vi "String - Format to (HH_colon_MM).vi"(10 "upper limit (Default 23 Hours)":i32=23, 11 "xx:xx":string) -> (2 "seconds":dbl format="%<%H:%M>t", 3 "(HH:mm)":string)   [LabVIEW 2013]
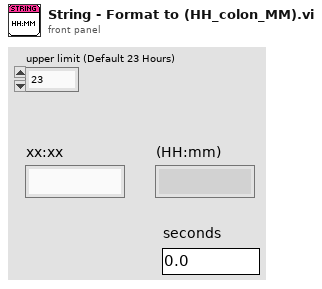
[diagram p1: front panel]
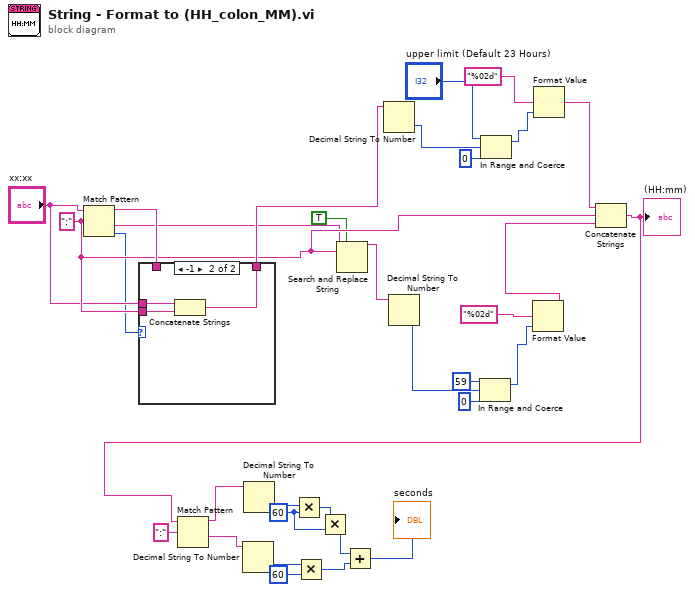
[diagram p0: block diagram]
diagram:
  w5 = 60 ("y")
  w30 = ":" ("regular expression")
  n1 = Match Pattern(string="xx:xx", regular expression=w30) -> (before substring=w31:string, after substring=w13:string, offset past match=w28:i32)  [unwired: 1 in, 1 out]
  n2 = case shown="-1" w28 {
    tunnel: "xx:xx" -> [_ w36]
    tunnel: w30 -> [_ w35]
    tunnel: w31 -> [w33 _]
    tunnel: [w33 w34] -> w32
    frame 0, Default {
    }
    frame -1 {
      n3 = Concatenate Strings(w36, w35) -> (w34:string)
    }
  }
  n4 = Search and Replace String(replace all?=TRUE ("replace all? (F)"), input string=w13, search string=w30) -> (result string=w15:string)  [unwired: 5 in, 3 out]
  n5 = Decimal String To Number(string=w32) -> (number=w26:i32)  [unwired: 2 in, 1 out]
  n6 = Decimal String To Number(string=w15) -> (number=w16:i32)  [unwired: 2 in, 1 out]
  n7 = In Range and Coerce(upper limit=59, x=w16, lower limit=0) -> (coerced(x)=w19:i32)  [unwired: 1 out]
  n8 = In Range and Coerce(upper limit="upper limit (Default 23 Hours)", x=w26, lower limit=0) -> (coerced(x)=w23:i32)  [unwired: 1 out]
  n9 = Format Value(format string="%02d", value (0)=w19) -> (output string=w20:string)  [unwired: 1 in]
  n10 = Format Value(format string="%02d", value (0)=w23) -> (output string=w27:string)  [unwired: 1 in]
  n11 = Concatenate Strings(w27, w30, w20) -> (w1:string)
  "(HH:mm)" <- w1
  n12 = Match Pattern(string=w1, regular expression=":") -> (before substring=w8:string, after substring=w11:string)  [unwired: 1 in, 2 out]
  n13 = Decimal String To Number(string=w11) -> (number=w10:i32)  [unwired: 2 in, 1 out]
  n14 = Decimal String To Number(string=w8) -> (number=w7:i32)  [unwired: 2 in, 1 out]
  n15 = Multiply(x=w7, y=w5) -> (x*y=w6:i32)
  n16 = Multiply(x=w10, y=60) -> (x*y=w3:i32)
  n17 = Multiply(x=w6, y=w5) -> (x*y=w4:i32)
  n18 = Add(x=w4, y=w3) -> (x+y=→"seconds":i32)
